vi "Read Live Report.vi"(8 "error in (no error)":errorcluster, 11 "TDMS in":refnum<class "TDMS.lvclass">) -> (0 "error out":errorcluster, 3 "TDMS out":refnum<class "TDMS.lvclass">)   [LabVIEW 2019, in "TDMS.lvlib" / "TDMS.lvclass"]
uses:
  TDMS.lvclass
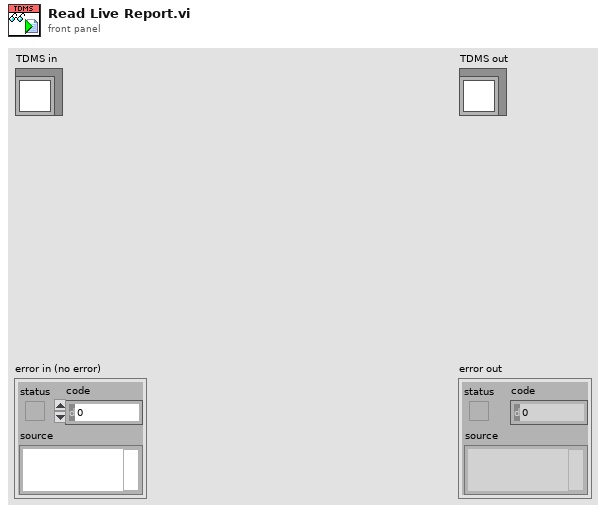
[diagram p1: front panel]
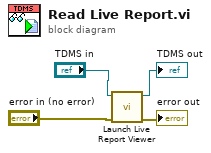
[diagram p0: block diagram]
diagram:
  n1 = call-dynamic "Launch Live Report Viewer.vi"("error in"="error in (no error)", "TDMS in"="TDMS in") -> ("error out"=→"error out":errorcluster, "TDMS out"=→"TDMS out":refnum<class "TDMS.lvclass">)  [unwired: 8 in]
